vi "myRIOXB DeviceCodeToName.vi"(9 "FullName?":bool, 11 "Device Code":string) -> (2 "Name":string)   [LabVIEW 2021]
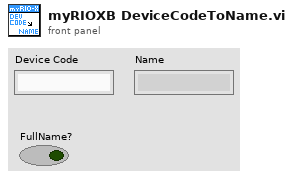
[diagram p1: front panel]
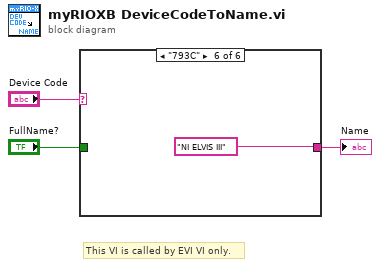
[diagram p0: block diagram]
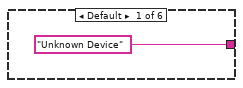
[diagram p2: hidden frame]
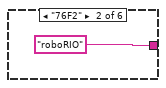
[diagram p3: hidden frame]
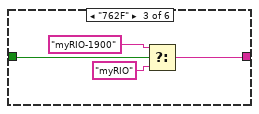
[diagram p4: hidden frame]
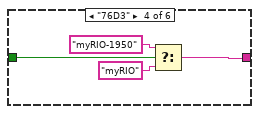
[diagram p5: hidden frame]
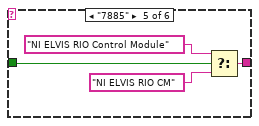
[diagram p6: hidden frame]
diagram:
  # "This VI is called by EVI VI only."
  n1 = case shown="\"793C\"" "Device Code" {
    tunnel: ["Unknown Device" "roboRIO" w7 w11 w15 "NI ELVIS III"] -> w2
    tunnel: "FullName?" -> [_ _ w6 w10 w14 _]
    frame Default {
    }
    frame "76F2" {
    }
    frame "762F" {
      n2 = Select(t="myRIO-1900", s=w6, f="myRIO") -> (s? t:f=w7:string)
    }
    frame "76D3" {
      n3 = Select(t="myRIO-1950", s=w10, f="myRIO") -> (s? t:f=w11:string)
    }
    frame "7885" {
      n4 = Select(t="NI ELVIS RIO Control Module", s=w14, f="NI ELVIS RIO CM") -> (s? t:f=w15:string)
    }
    frame "793C" {
    }
  }
  "Name" <- w2
